vi "Belkin Globals.vi"() -> ()   [LabVIEW 2015]
panel:
  out "ActualUppervalue":sgl
  out "max index(es)":i32
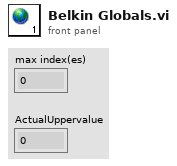
[diagram p1: front panel]
diagram:
